vi "数字至ASCII码字符转换.vi"(3 "数字":i32) -> (0 "ASCII码字符串":string)   [LabVIEW 8.6]
panel:
  out "偶数长度十六进制字符串":string
  out "十六进制数组":i32[](array[numeric])
  out "十六进制整型字符串":string
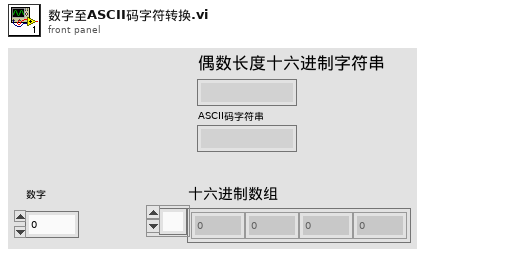
[diagram p1: front panel]
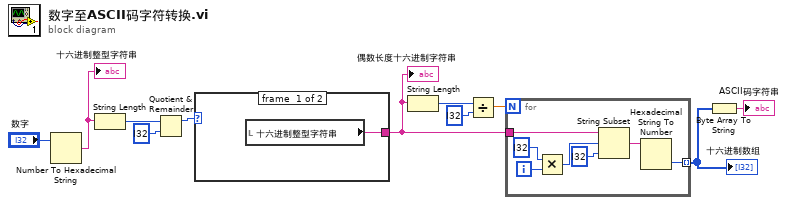
[diagram p0: block diagram]
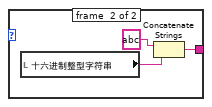
[diagram p2: hidden frame]
diagram:
  n1 = Number To Hexadecimal String(2:"数字") -> (0:w11:string)  [unwired: 1 in]
  "十六进制整型字符串" <- w11
  n2 = String Length(string=w11) -> (length=w8:i32)
  n3 = Quotient & Remainder(x=w8, y=i32 ?) -> (x-y*floor(x/y)=w9:i32)  [unwired: 1 out]
  n4 = case shown="1" w9 {
    tunnel: [w12 w15] -> w7
    frame #0 {
      n5 = local read "十六进制整型字符串"() -> (w12:string)
    }
    frame #1 {
      n6 = local read "十六进制整型字符串"() -> (w13:string)
      n7 = Concatenate Strings(string ?, w13) -> (w15:string)
    }
  }
  "偶数长度十六进制字符串" <- w7
  n8 = String Length(string=w7) -> (length=w6:i32)
  n9 = Divide(x=w6, y=i32 ?) -> (x/y=w4:dbl)
  n10 = for {
    N: w4 -> [_]
    tunnel: w7 -> [w22]
    tunnel: [w16] -> w2 mode=indexing
    i -> [w21]
    n11 = Multiply(x=i32 ?, y=w21) -> (x*y=w19:i32)
    n12 = String Subset(string=w22, offset (0)=w19, length (rest)=i32 ? ("长度（剩余）")) -> (substring=w17:string)
    n13 = Hexadecimal String To Number(string=w17) -> (number=w16:u32)  [unwired: 2 in, 1 out]
  }
  "十六进制数组" <- w2
  n14 = Byte Array To String(unsigned byte array=w2) -> (string=→"ASCII码字符串":string)
